vi "FG VFH Motor Command.vi"(2 "FG Action":T2, 3 "Motor Command in":T1) -> (1 "Motor Command out":T1)   [LabVIEW 2009]
uses:
  Actions for FG's.ctl
  Remote Control/Motor Command.ctl
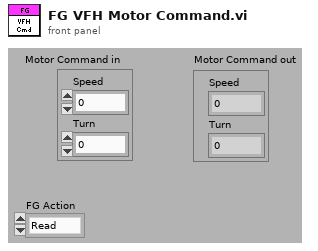
[diagram p1: front panel]
types:
  T1 = typedef "Motor Command.ctl" = cluster{"Speed":i16, "Turn":i16}
  T2 = typedef "Actions for FG's.ctl" = enum16{"Read", "Write"}
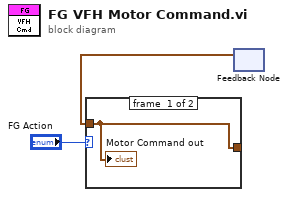
[diagram p0: block diagram]
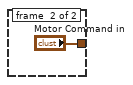
[diagram p2: hidden frame]
diagram:
  n1 = feedback #1() -> (w1:T1)  [unwired: 1 in]
  n2 = case shown="\"Read\", Default" "FG Action" {
    tunnel: [w4 "Motor Command in"] -> w2
    tunnel: w1 -> [w4 _]
    frame #0 {
      "Motor Command out" <- w4
    }
    frame #1 {
    }
  }
